vi "Initialize Plugin.vi"(7 "id":i32, 8 "error in (no error)":errorcluster, 10 "Buffers":refnum<class "Buffers.lvclass">, 11 "Plugin Configuration":T1={"name"="", "class"="", "cycle timing"={"priority"=0, "decimation"=1, "offset"=0}, "Transfer Groups"=[], "settings"=[], "thread count"=0} {"Transfer Groups"."Transfers"."channels"."dst buffer offset" format="%d bytes"; "Transfer Groups"."Transfers"."channels"."src buffer offset" format="%d bytes"}) -> (0 "error out":errorcluster, 3 "Plugin out":refnum<class "Plugin.lvclass">)   [LabVIEW 2017, in "DSF Core.lvlib" / "Plugin.lvclass"]
uses:
  Plugin.lvclass
  Transfer Group/Transfer Group.lvclass
  DSF Core.lvlib
  DSF Configuration API/Public/Required Buffer Size (Transfer Group).vi
  Debug/Debug Flags/Debug Flags.lvclass
  DSF Configuration API/Public/Controls/DSF Timing Info.ctl
  DSF Configuration API/Public/Controls/DSF Direction.ctl
  DSF Configuration API/Public/Controls/DSF Byte Order.ctl
  DSF Configuration API/Public/Controls/DSF Data Type.ctl
  DSF Configuration API/Public/Controls/DSF Settings Info.ctl
  DSF Configuration API/Public/Controls/DSF Engine Channel Configuration.ctl
  DSF Configuration API/Public/Controls/DSF Engine Transfer Configuration.ctl
  DSF Configuration API/Public/Controls/DSF Engine Transfer Group Configuration.ctl
  DSF Configuration API/Public/Controls/DSF Engine Plugin Configuration.ctl
  Buffer/Buffers.lvclass
panel:
  in  "component classes":refnum<class>[](array[class])
  in  "Debug Flags":refnum<class "Debug Flags.lvclass">
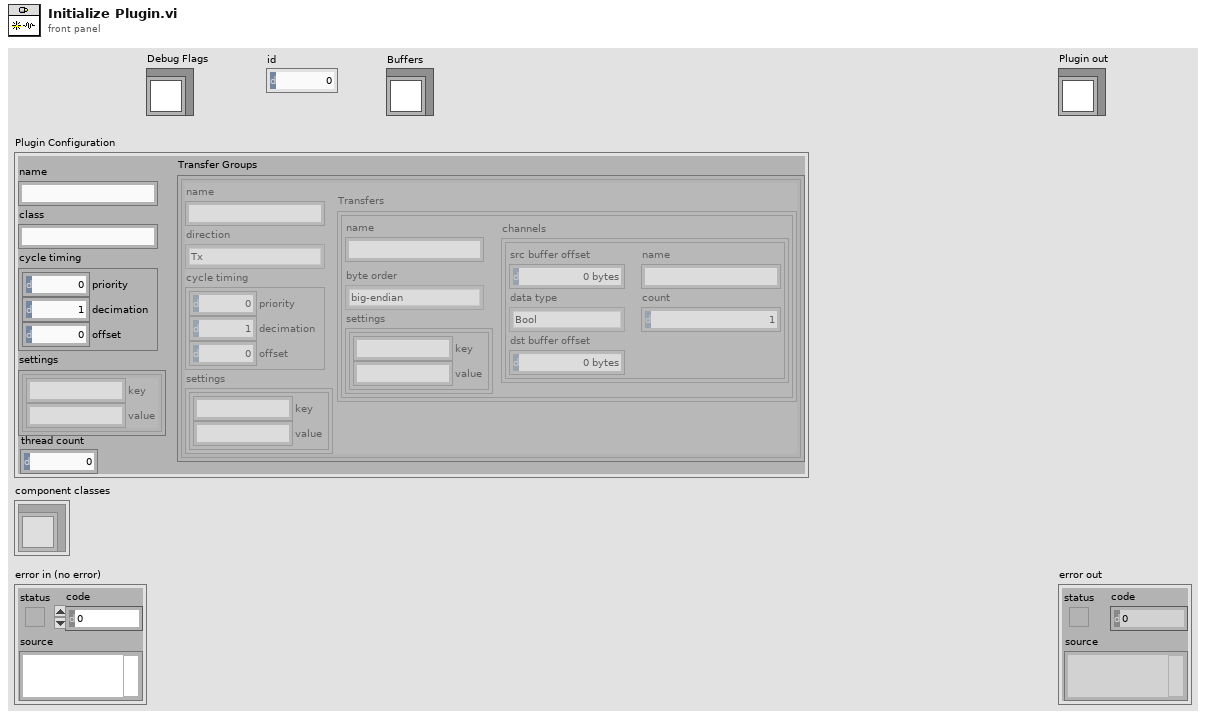
[diagram p1: front panel]
types:
  T1 = typedef "DSF Core.lvlib/DSF Engine Plugin Configuration.ctl" = cluster{"name":string, "class":string, "cycle timing":T2, "Transfer Groups":T3[], "settings":T9, "thread count":i32}
  T2 = typedef "DSF Core.lvlib/DSF Timing Info.ctl" = cluster{"priority":u64, "decimation":u64, "offset":u64}
  T3 = typedef "DSF Core.lvlib/DSF Engine Transfer Group Configuration.ctl" = cluster{"name":string, "direction":T4, "cycle timing":T2, "Transfers":T5[], "settings":T9}
  T4 = typedef "DSF Core.lvlib/DSF Direction.ctl" = enum8{"Tx", "Rx"}
  T5 = typedef "DSF Core.lvlib/DSF Engine Transfer Configuration.ctl" = cluster{"name":string, "byte order":T6, "channels":T7[], "settings":T9}
  T6 = typedef "DSF Core.lvlib/DSF Byte Order.ctl" = enum8{"big-endian", "little-endian"}
  T7 = typedef "DSF Core.lvlib/DSF Engine Channel Configuration.ctl" = cluster{"src buffer offset":u64, "name":string, "data type":T8, "count":u64, "dst buffer offset":u64}
  T8 = typedef "DSF Core.lvlib/DSF Data Type.ctl" = enum8{"Bool", "SGL", "DBL", "I8", "I16", "I32", "I64", "U8", "U16", "U32", "U64"}
  T9 = typedef "DSF Core.lvlib/DSF Settings Info.ctl" = cluster{"key":string, "value":string}[]
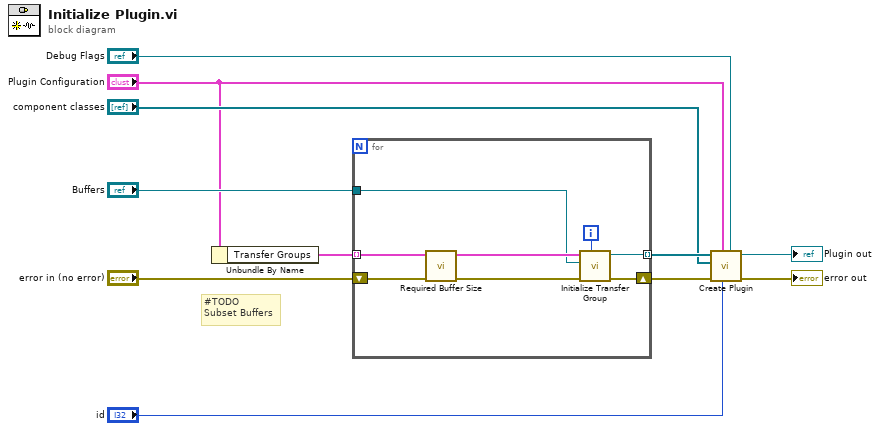
[diagram p0: block diagram]
diagram:
  # "#TODO\nSubset Buffers"
  n1 = Unbundle By Name("Plugin Configuration") -> ("Transfer Groups"=w11:T3[])
  n2 = for {
    tunnel: w11 -> [w16] mode=indexing
    shift-right: [w19] -> w9
    shift-left: "error in (no error)" -> [w14]
    tunnel: [w18] -> w10 mode=indexing
    tunnel: "Buffers" -> [w12]
    i -> [w17]
    n3 = call-poly "Required Buffer Size.vi"("error in (no error)"=w14, "Transfer Group Configuration in"=w16) -> ("error out"=w13:errorcluster, "Transfer Group Configuration out"=w15:T3)  [unwired: 7 in, 1 out]
    n4 = call "Initialize Transfer Group.vi"("id"=w17, "error in (no error)"=w13, "Buffers"=w12, "Transfer Group Configuration"=w15) -> ("error out"=w19:errorcluster, "Transfer Group out"=w18:refnum<class "Transfer Group.lvclass">)  [unwired: 6 in]
  }
  n5 = call "Create Plugin.vi"("Debug Flags"="Debug Flags", "framework id"="id", "Plugin Configuration"="Plugin Configuration", "error in (no error)"=w9, "component classes"="component classes", "Transfer Groups"=w10) -> ("error out"=→"error out":errorcluster, "Plugin out"=→"Plugin out":refnum<class "Plugin.lvclass">)  [unwired: 4 in]
